vi "finishPassToStrikerPlay.vi"(8 "error in (no error)":errorcluster, 10 "Game":refnum<class "Game.lvclass">, 11 "PassToStriker in":refnum<class "PassToStriker.lvclass">) -> (0 "error out":errorcluster, 2 "result":bool, 3 "PassToStriker out":refnum<class "PassToStriker.lvclass">)   [LabVIEW 2023, in "PassToStriker.lvclass"]
uses:
  PassToStriker.lvclass
  Game_class/Game.lvclass
  Referee_class/command_interpreted.ctl
  Game_class/Game.lvclass/Game.ctl
  Referee_class/Referee.lvclass/Referee.ctl
  Events_class/Events.lvclass/Events.ctl
  Game_class/Read EventsRef.vi
  Events_class/Read touch.vi
  Events_class/Read id_touch.vi
  Events_class/Read ball_out.vi
  Game_class/Read Referee.vi
  Referee_class/Read command_interpreted.vi
  Referee_class/Referee.lvclass
  Events_class/Events.lvclass
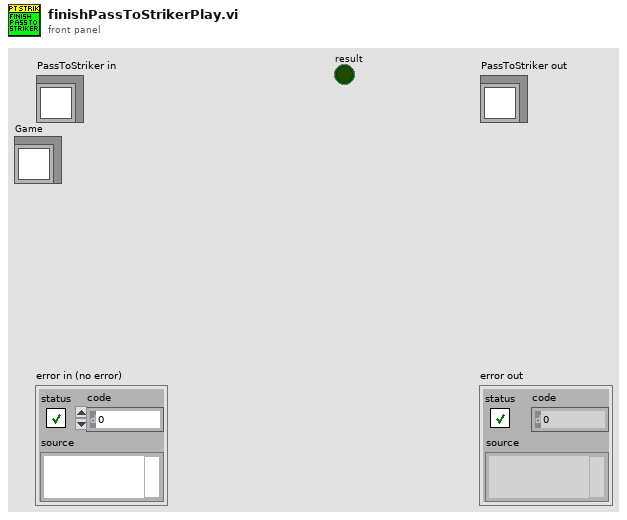
[diagram p1: front panel]
types:
  T1 = typedef "command_interpreted.ctl" = enum16{"Goal Ally", "Goal Enemy", "Ball Placement Enemy", "Ball Placement Ally", "Normal Half Time", "Extra Time  Break", "Extra Half Time", "None", "Post Game", "PKA Normal Start", "Prepare Kickoff Ally", "PKE Normal Start", "Prepare Kickoff Enemy", "Force Start", "Halt", "Timeout", "Prepare Penalty Ally", "Prepare Penalty Enemy", "PPA NormalStart", "PPE Normal Start", "Indirect Free Ally", "Direct Free Enemy", "Direct Free Ally", "Indirect Free Enemy", "Stop"}
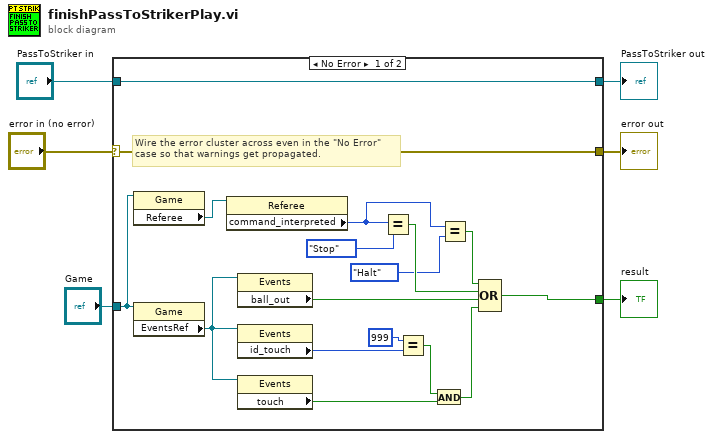
[diagram p0: block diagram]
diagram:
  n1 = case shown="No Error" "error in (no error)" {
    selector: "error in (no error)" -> [w22 w25]
    tunnel: [w22 w25] -> w5
    tunnel: [w23 w24] -> w3
    tunnel: "PassToStriker in" -> [w23 w24]
    tunnel: [w13 _] -> w2
    tunnel: "Game" -> [w12 _]
    frame No Error {
      # "Wire the error cluster across even in the \"No Error\"\ncase so that warnings get propagated."
      n2 = property class="Game"(reference=w12) -> ("Referee"=w15:refnum<class "Referee.lvclass">)  [unwired: 1 in, 2 out]
      n3 = property class="Game"(reference=w12) -> ("EventsRef"=w21:refnum<class "Events.lvclass">)  [unwired: 1 in, 2 out]
      n4 = property class="Referee"(reference=w15) -> ("command_interpreted"=w9:T1)  [unwired: 1 in, 2 out]
      n5 = property class="Events"(reference=w21) -> ("ball_out"=w18:bool)  [unwired: 1 in, 2 out]
      n6 = property class="Events"(reference=w21) -> ("id_touch"=w19:i32)  [unwired: 1 in, 2 out]
      n7 = property class="Events"(reference=w21) -> ("touch"=w14:bool)  [unwired: 1 in, 2 out]
      n8 = Equal?(x=w9, y=command_interpreted."Stop") -> (x = y?=w10:bool)
      n9 = Equal?(x=999 ("id_touch"), y=w19) -> (x = y?=w17:bool)
      n10 = And(x=w17, y=w14) -> (x .and. y?=w16:bool)
      n11 = Equal?(x=w9, y=command_interpreted."Halt") -> (x = y?=w7:bool)
      n12 = Compound Arithmetic op=OR(w7, w10, w18, w16) -> (w13:bool)
    }
    frame Error {
    }
  }
  "error out" <- w5
  "PassToStriker out" <- w3
  "result" <- w2
